vi "Write Data.vi"(8 "Error In":errorcluster, 10 "Data":cluster{"Key":string, "Value":variant}[](array[cluster]), 11 "Non-Terminal In":refnum<class "NonTerminal.lvclass">) -> (0 "Error Out":errorcluster, 3 "Non-Terminal Out":refnum<class "NonTerminal.lvclass">)   [LabVIEW 2018, in "Toolkit.lvlib" / "Nodes.lvlib" / "NonTerminal.lvclass"]
uses:
  NonTerminal.lvclass
  NonTerminal.lvclass/NonTerminal.ctl
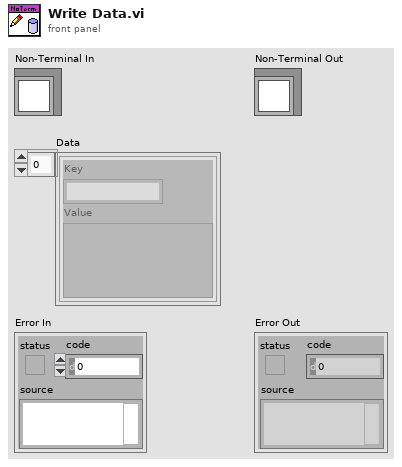
[diagram p1: front panel]
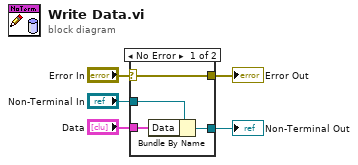
[diagram p0: block diagram]
diagram:
  n1 = case shown="No Error" "Error In" {
    selector: "Error In" -> [w9 w10]
    tunnel: [w9 w10] -> w4
    tunnel: [w7 w11] -> w2
    tunnel: "Non-Terminal In" -> [w8 w11]
    tunnel: "Data" -> [w6 _]
    frame No Error {
      n2 = Bundle By Name(cluster=w8, "Data"=w6) -> (w7:refnum<class "NonTerminal.lvclass">)
    }
    frame Error {
    }
  }
  "Error Out" <- w4
  "Non-Terminal Out" <- w2
